vi "VNA.vi"() -> ()   [LabVIEW 2022 SP3]
uses:
  <instrlib>/Agilent ENA Series/Agilent ENA Series.lvlib
  <vilib>/Utility/file.llb/Write Delimited Spreadsheet (DBL).vi
panel:
  out "Waveform Graph":dbl[](graph)
  in  "Safe Mode Maximum Power Level (30)":dbl=30.0
  in  "Safe Mode Minimum Power Level (-200)":dbl=-200.0
  in  "Tolerance Level (5)":dbl=5.0
  in  "Power Level Offset (0)":dbl
  in  "Port ( 1)":i32=1
  in  "Channel (1)":i32=1
  in  "Enable Safe Mode (T: Enabled)":bool=TRUE
  in  "Enable Receiver Leveling (T: Enabled)":bool=TRUE
  in  "Reset? (T: Yes)":bool=TRUE
  in  "ID Query? (T: Yes)":bool=TRUE
  out "High":dbl
  out "Low":dbl
  out "Center Frequency":dbl format="%^.2e"
  out "Q Value":dbl format="%^.2e"
  out "Loss":dbl format="%^.2e"
  out "Bandwidth":dbl format="%^.2e"
  in  "VISA resource name":refnum<visa-resource-name>
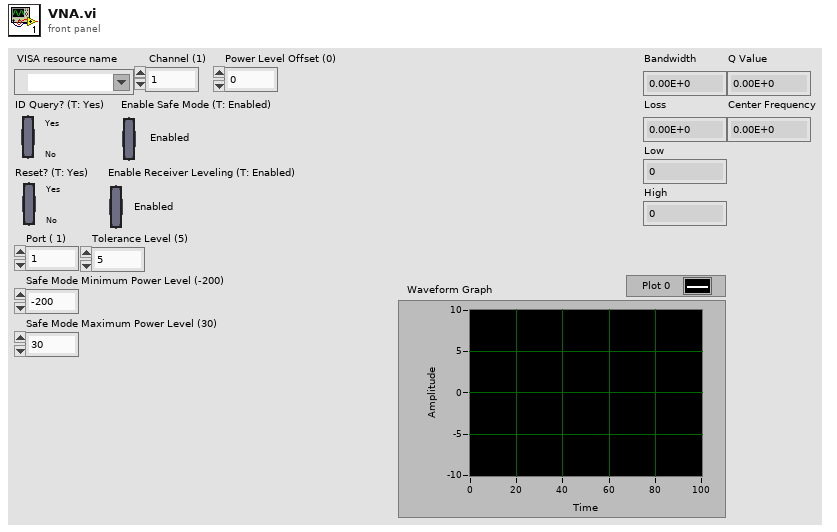
[diagram p1: front panel]
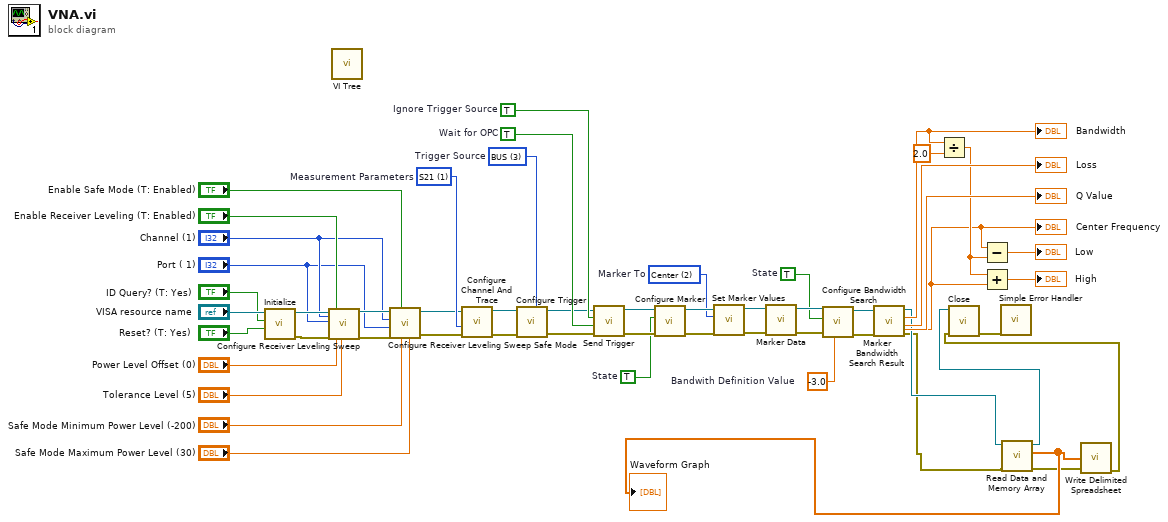
[diagram p0: block diagram]
diagram:
  w23 = u16 1 items=["S11", "S21", "S31", "S41", "S12", "S22", "S32", "S42", "S13", "S23", "S33", "S43", "S14", "S24", "S34", "S44", "A", "B", "C", "D", "R1", "R2", "R3", "R4"]  # Measurement Parameters
  w40 = -3.0  # Bandwith Definition Value
  w41 = TRUE  # State
  w46 = u16 2 items=["Start", "Stop", "Center", "Reference", "Electrical Delay"]  # Marker To
  w49 = TRUE  # State
  w52 = TRUE  # Wait for OPC
  w53 = TRUE  # Ignore Trigger Source
  w54 = u16 3 items=["Internal", "External", "Manual", "BUS"]  # Trigger Source
  n1 = call <instrlib>:"Initialize.vi"("Reset? (T: Yes)"="Reset? (T: Yes)", "ID Query? (T: Yes)"="ID Query? (T: Yes)", "VISA resource name"="VISA resource name") -> ("error out"=w21:errorcluster, "VISA resource name out"=w22:refnum<visa-resource-name>)  [unwired: 7 in]
  n2 = call <instrlib>:"Configure Receiver Leveling Sweep.vi"("VISA resource name"=w22, "Channel (1)"="Channel (1)", "Port ( 1)"="Port ( 1)", "error in (no error)"=w21, "Enable Receiver Leveling (F: Disabled)"="Enable Receiver Leveling (T: Enabled)", "Power Level Offset (0)"="Power Level Offset (0)", "Tolerance Level (5)"="Tolerance Level (5)") -> ("VISA resource name out"=w16:refnum<visa-resource-name>, "error out"=w15:errorcluster)  [unwired: 11 in]
  n3 = call <instrlib>:"VI Tree.vi"() -> ()  [unwired: 12 in]
  n4 = call <instrlib>:"Configure Receiver Leveling Sweep Safe Mode.vi"("Safe Mode Maximum Power Level (30)"="Safe Mode Maximum Power Level (30)", "Safe Mode Minimum Power Level (-200)"="Safe Mode Minimum Power Level (-200)", "Enable Safe Mode (F: Disabled)"="Enable Safe Mode (T: Enabled)", "error in (no error)"=w15, "Port ( 1)"="Port ( 1)", "Channel (1)"="Channel (1)", "VISA resource name"=w16) -> ("error out"=w19:errorcluster, "VISA resource name out"=w20:refnum<visa-resource-name>)  [unwired: 3 in]
  n5 = call <instrlib>:"Configure Channel And Trace.vi"("error in (no error)"=w19, "Measurement Parameters (0: S11)"=w23, "VISA resource name"=w20) -> ("error out"=w17:errorcluster, "VISA resource name out"=w18:refnum<visa-resource-name>)  [unwired: 7 in]
  n6 = call <instrlib>:"Configure Trigger.vi"("Trigger Source (0: Internal)"=w54, "error in (no error)"=w17, "VISA resource name"=w18) -> ("error out"=w24:errorcluster, "VISA resource name out"=w25:refnum<visa-resource-name>)  [unwired: 7 in]
  n7 = call <instrlib>:"Send Trigger.vi"("error in (no error)"=w24, "Wait for OPC (F: Do not Wait)"=w52, "Ignore Trigger Source (F: Do not Ignore)"=w53, "VISA resource name"=w25) -> ("error out"=w50:errorcluster, "VISA resource name out"=w51:refnum<visa-resource-name>)  [unwired: 6 in]
  n8 = call <instrlib>:"Configure Marker.vi"("error in (no error)"=w50, "Marker State (F: Disabled)"=w49, "VISA resource name"=w51) -> ("error out"=w47:errorcluster, "VISA resource name out"=w48:refnum<visa-resource-name>)  [unwired: 7 in]
  n9 = call <instrlib>:"Set Marker Values.vi"("error in (no error)"=w47, "Marker To (0: Start)"=w46, "VISA resource name"=w48) -> ("error out"=w44:errorcluster, "VISA resource name out"=w45:refnum<visa-resource-name>)  [unwired: 7 in]
  n10 = call <instrlib>:"Marker Data.vi"("error in (no error)"=w44, "VISA resource name"=w45) -> ("error out"=w42:errorcluster, "VISA resource name out"=w43:refnum<visa-resource-name>)  [unwired: 5 in, 3 out]
  n11 = call <instrlib>:"Configure Bandwidth Search.vi"("Bandwidth Definition Value (-3.0)"=w40, "error in (no error)"=w42, "Result Display State (F: Disable)"=w41, "VISA resource name"=w43) -> ("error out"=w38:errorcluster, "VISA resource name out"=w39:refnum<visa-resource-name>)  [unwired: 6 in]
  n12 = call <instrlib>:"Marker Bandwidth Search Result.vi"("error in (no error)"=w38, "VISA resource name"=w39) -> ("error out"=w4:errorcluster, "Loss"=→"Loss":dbl, "Bandwidth"=w35:dbl, "VISA resource name out"=w6:refnum<visa-resource-name>, "Q Value"=→"Q Value":dbl, "Center Frequency"=w31:dbl)  [unwired: 4 in]
  "Bandwidth" <- w35
  "Center Frequency" <- w31
  n13 = Divide(x=w35, y=2.0) -> (x/y=w32:dbl)
  n14 = Subtract(x=w31, y=w32) -> (x-y=→"Low":dbl)
  n15 = Add(x=w32, y=w31) -> (x+y=→"High":dbl)
  n16 = call <instrlib>:"Read Data and Memory Array.vi"("error in (no error)"=w4, "VISA resource name"=w6) -> ("error out"=w3:errorcluster, "Primary / Real"=w5:dbl[], "VISA resource name out"=w1:refnum<visa-resource-name>)  [unwired: 6 in, 1 out]
  "Waveform Graph" <- w5
  n17 = call-poly <vilib>:"Write Delimited Spreadsheet.vi"("1D data"=w5, "error in (no error)"=w3) -> ("error out"=w2:errorcluster)  [unwired: 12 in, 1 out]
  n18 = call <instrlib>:"Close.vi"("error in (no error)"=w2, "VISA resource name"=w1) -> ("error out"=w29:errorcluster)  [unwired: 9 in]
  n19 = call <vilib>:"Simple Error Handler.vi"("error in (no error)"=w29) -> ()  [unwired: 4 in, 5 out]
